vi "tec_ctl_params.vi"(6 "DevID":string, 7 "LVWSR":refnum<class "Web Request.lvclass">, 9 "d":dbl, 10 "i":dbl, 11 "p":dbl) -> ()   [LabVIEW 2014]
uses:
  <vilib>/wsapi/Web Request.lvclass
  Controller/Messages/Update TE Tech PID/Update TEC PID.lvclass
  Controller/Messages/Update TE Tech PID/Update TEC PID.lvclass/Update TEC PID.ctl
  Controller/Messages/Update TE Tech PID/Write DevID.vi
  Controller/Messages/Update TE Tech PID/Write ctl.vi
  Controller/Controller.lvclass
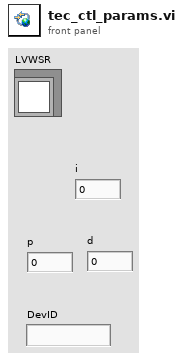
[diagram p1: front panel]
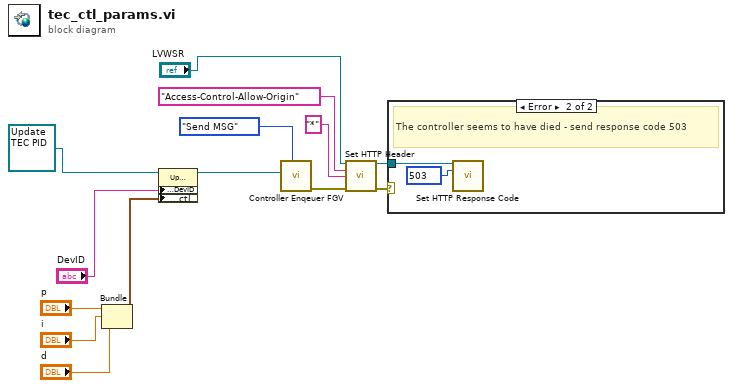
[diagram p0: block diagram]
diagram:
  n1 = Bundle("p"="p", "i"="i", "d"="d") -> (w1:cluster{"p":dbl, "i":dbl, "d":dbl})  [unwired: 1 in]
  n2 = property class="Update TEC PID.lvclass"(reference=refnum<class "Update TEC PID.lvclass"> refnum ("Controller:Update TEC PID.lvclass"), "Accessors:DevID"="DevID", "Accessors:ctl"=w1) -> (reference out=w9:refnum<class "Update TEC PID.lvclass">)  [unwired: 1 in, 1 out]
  n3 = call "Controller Enqeuer FGV.vi"("State"=enum16{"Store", "Send MSG"}."Send MSG", "MSG"=w9) -> ("error out"=w8:errorcluster)  [unwired: 9 in]
  n4 = call <vilib>:"Set HTTP Header.vi"("LabVIEW Web Service Request"="LVWSR", "header"="Access-Control-Allow-Origin", "header value"="*", "error in (no error)"=w8) -> ("LabVIEW Web Service Request out"=w12:refnum<class "Web Request.lvclass">, "error out"=w11:errorcluster)  [unwired: 10 in]
  n5 = case shown="Error" w11 {
    tunnel: w12 -> [_ w15]
    frame No Error {
    }
    frame Error {
      w16 = 503 items=["100"=100, "101"=101, "200"=200, "201"=201, "202"=202, "203"=203, "204"=204, "205"=205, "206"=206, "300"=300, "301"=301, "302"=302, "303"=303, "304"=304, "305"=305, "306"=306, "307"=307, "400"=400, "401"=401, "402"=402, "403"=403, "404"=404, "405"=405, "406"=406, "407"=407, "408"=408, "409"=409, "410"=410, "411"=411, "412"=412, "413"=413, "414"=414, "415"=415, "416"=416, "417"=417, "500"=500, "501"=501, "502"=502, "503"=503, "504"=504, "505"=505] ("response code (200)")
      # "The controller seems to have died - send response code 503"
      n6 = call <vilib>:"Set HTTP Response Code.vi"("LabVIEW Web Service Request"=w15, "response code (200)"=w16) -> ()  [unwired: 12 in, 2 out]
    }
  }
